vi "AO config UI to not UI.vi"(10 "output terminal configuration":i32(ring)=-1 items=["Default"=-1, "RSE"=10083, "Differential"=10106, "Pseudodifferential"=12529], 11 "AO Config (UI)":T1) -> (3 "AO Config":T4 {"output terminal configuration" items=["Default"=-1, "RSE"=10083, "Differential"=10106, "Pseudodifferential"=12529]})   [LabVIEW 2016, in "Instrument.Lockin.lvclass"]
uses:
  Instrument.Lockin.lvclass
  LockinDAQ/Typedefs/446xAO-enum.ctl
  LockinDAQ/LockinDAQ.lvclass
  LockinDAQ/Typedefs/DAQType-enum.ctl
  LockinDAQ/Typedefs/AO.config-cluster.ctl
  LockinDAQ/Typedefs/AO.config(UI)-cluster.ctl
  LockinDAQ/Typedefs/AO.config(UI)-array.ctl
  LockinDAQ/Typedefs/AO.config-array.ctl
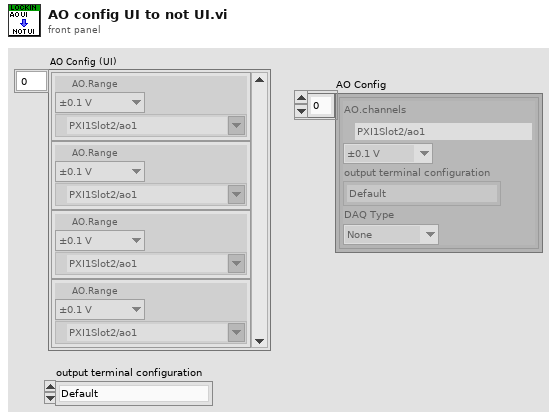
[diagram p1: front panel]
types:
  T1 = typedef "LockinDAQ.lvclass/AO.config(UI)-array.ctl" = T2[]
  T2 = typedef "LockinDAQ.lvclass/AO.config(UI)-cluster.ctl" = cluster{"AO.Range":T3, "AO.channels":tag}
  T3 = typedef "LockinDAQ.lvclass/446xAO-enum.ctl" = enum16{"±0.1 V", "±1.0 V", "±10.0 V"}
  T4 = typedef "LockinDAQ.lvclass/AO.config-array.ctl" = T5[]
  T5 = typedef "LockinDAQ.lvclass/AO.config-cluster.ctl" = cluster{"AO.channels":tag, "AO.Range":T3, "output terminal configuration":i32, "DAQ Type":T6}
  T6 = typedef "LockinDAQ.lvclass/DAQType-enum.ctl" = enum16{"None", "USB 4431", "PXI 446x"}
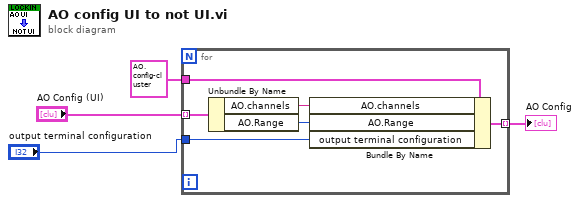
[diagram p0: block diagram]
diagram:
  n1 = for {
    tunnel: T5 {"AO.channels"="PXI1Slot2/ao1", "AO.Range"=enum."±0.1 V", "output terminal configuration"=-1, "DAQ Type"=enum."None"} ("AO.config") -> [w10]
    tunnel: "AO Config (UI)" -> [w9] mode=indexing
    tunnel: [w6] -> w4 mode=indexing
    tunnel: "output terminal configuration" -> [w5]
    n2 = Unbundle By Name(w9) -> ("AO.channels"=w8:tag, "AO.Range"=w7:T3)
    n3 = Bundle By Name(cluster=w10, "AO.channels"=w8, "AO.Range"=w7, "output terminal configuration"=w5) -> (w6:T5)
  }
  "AO Config" <- w4
